vi "Scale Image.vi"() -> ()   [LabVIEW 2018]
doc: "Scale Image: This example is a scaling image example, which can change the size of the image, scaling proportionally or non proportionally. Scaling proportionally means that both width and height are scaled to the same ratio to maintain the same aspect ratio of the image."
uses:
  vi.lib/VIRobotics/opencv_yiku/ctls/ColorConversionCodes.ctl
  vi.lib/VIRobotics/opencv_yiku/Mat/Mat_8U/Mat_8U.lvclass
  D:/Program Files/company/National Instruments/LabVIEW 2018/vi.lib/addons/VIRobotics/opencv_yiku/Mat/Mat/Mat.lvclass
  vi.lib/VIRobotics/opencv_yiku/Mat/Create_Mat_8U.vi
  vi.lib/VIRobotics/opencv_yiku/opencv_yiku.lvlib
panel:
  out "resized_img 2":picture
  out "resized_img":picture
  out "img":picture
  # "Overview: Demonstrates how to resize the image.\nRequirements: Windows.\nInstructions: \n1. Run the VI"
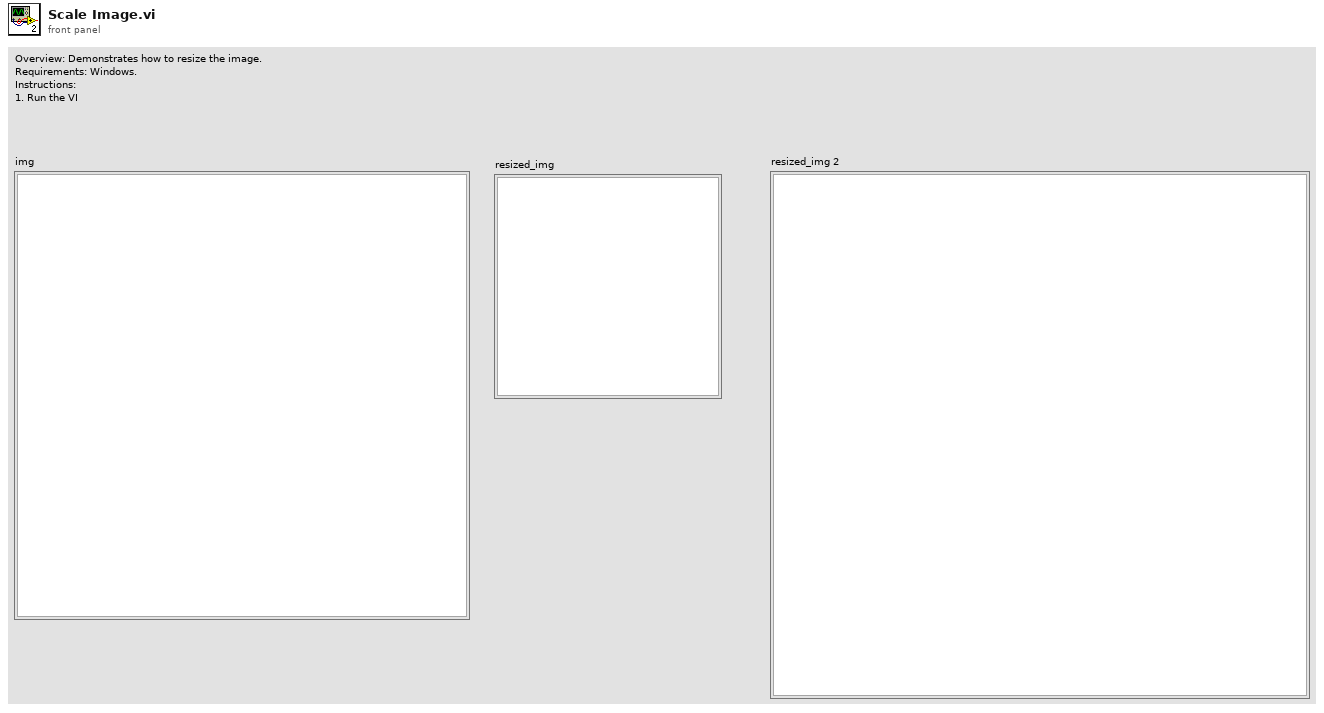
[diagram p1: front panel]
types:
  T1 = typedef "opencv_yiku.lvlib/ColorConversionCodes.ctl" = enum32{"COLOR_BGR2BGRA", "COLOR_BGRA2BGR", "COLOR_BGR2RGBA", "COLOR_RGBA2BGR", "COLOR_BGR2RGB", "COLOR_BGRA2RGBA", "COLOR_BGR2GRAY", "COLOR_RGB2GRAY", "COLOR_GRAY2BGR", "COLOR_GRAY2BGRA", "COLOR_BGRA2GRAY", "COLOR_RGBA2GRAY", "COLOR_BGR2BGR565", "COLOR_RGB2BGR565", "COLOR_BGR5652BGR", "COLOR_BGR5652RGB", "COLOR_BGRA2BGR565", "COLOR_RGBA2BGR565", "COLOR_BGR5652BGRA", "COLOR_BGR5652RGBA", "COLOR_GRAY2BGR565", "COLOR_BGR5652GRAY", "COLOR_BGR2BGR555", "COLOR_RGB2BGR555", "COLOR_BGR5552BGR", "COLOR_BGR5552RGB", "COLOR_BGRA2BGR555", "COLOR_RGBA2BGR555", "COLOR_BGR5552BGRA", "COLOR_BGR5552RGBA", "COLOR_GRAY2BGR555", "COLOR_BGR5552GRAY", "COLOR_BGR2XYZ", "COLOR_RGB2XYZ", "COLOR_XYZ2BGR", "COLOR_XYZ2RGB", "COLOR_BGR2YCrCb", "COLOR_RGB2YCrCb", "COLOR_YCrCb2BGR", "COLOR_YCrCb2RGB", "COLOR_BGR2HSV", "COLOR_RGB2HSV", "42", "43", "COLOR_BGR2Lab", "COLOR_RGB2Lab"}
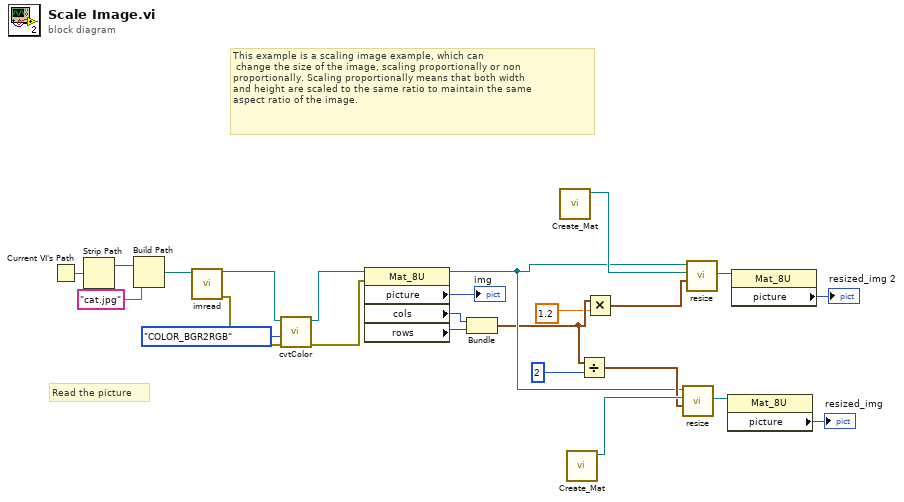
[diagram p0: block diagram]
diagram:
  # "This example is a scaling image example, which can\n change the size of the image, scaling proportionally or non \nproportionally. Scaling proportionally means that both width \nand height are scaled to the same ratio to maintain the same \naspect ratio of the image."
  # "Read the picture"
  n1 = Current VI's Path() -> (path=w22:path)
  n2 = Strip Path(path=w22) -> (stripped path=w24:path)  [unwired: 1 out]
  n3 = Build Path(base path=w24, name or relative path="cat.jpg") -> (appended path=w21:path)
  n4 = call "imread.vi"("path"=w21) -> ("error out"=w18:errorcluster, "Mat out"=w20:refnum<class "Mat_8U.lvclass">)  [unwired: 9 in]
  n5 = call "cvtColor.vi"("error in (no error)"=w18, "dstCn"=ColorConversionCodes."COLOR_BGR2RGB", "src"=w20) -> ("error out"=w17:errorcluster, "src out"=w19:refnum<class "Mat_8U.lvclass">)  [unwired: 6 in, 1 out]
  n6 = property class="Mat_8U"(reference=w19, error in=w17) -> (reference out=w5:refnum<class "Mat_8U.lvclass">, "picture"=→"img":picture, "cols"=w13:i32, "rows"=w12:i32)  [unwired: 1 out]
  n7 = Bundle("cols"=w13, "rows"=w12) -> (w4:cluster{"cols":i32, "rows":i32})  [unwired: 1 in]
  n8 = call-poly "Create_Mat.vi"() -> ("Mat_8U_out"=w8:refnum<class "Mat_8U.lvclass">)  [unwired: 10 in, 1 out]
  n9 = call-poly "Create_Mat.vi"() -> ("Mat_8U_out"=w14:refnum<class "Mat_8U.lvclass">)  [unwired: 10 in, 1 out]
  n10 = Divide(x=w4, y=2) -> (x/y=w11:cluster{"cols":dbl, "rows":dbl})
  n11 = Multiply(x=w4, y=1.2) -> (x*y=w2:cluster{"cols":dbl, "rows":dbl})
  n12 = call "resize.vi"("Size"=w11, "dst"=w14, "src"=w5) -> ("dst out"=w10:refnum<class "Mat_8U.lvclass">)  [unwired: 6 in, 2 out]
  n13 = call "resize.vi"("Size"=w2, "dst"=w8, "src"=w5) -> ("dst out"=w7:refnum<class "Mat_8U.lvclass">)  [unwired: 6 in, 2 out]
  n14 = property class="Mat_8U"(reference=w10) -> ("picture"=→"resized_img":picture)  [unwired: 1 in, 2 out]
  n15 = property class="Mat_8U"(reference=w7) -> ("picture"=→"resized_img 2":picture)  [unwired: 1 in, 2 out]
